vi "DataLog Merge Times.vi"(0 "times to add":dbl[](array[numeric]) format="%<%H:%M:%S%2u\n%Y/%m/%d>T", 7 "times in":dbl[](array[numeric]) format="%<%H:%M:%S%2u\n%Y/%m/%d>T", 11 "error in (no error)":errorcluster) -> (8 "times out":dbl[](array[numeric]) format="%<%H:%M:%S%2u\n%Y/%m/%d>T", 15 "error out":errorcluster)   [LabVIEW 2012]
doc: "Merge times for interpolation. Given two arrays of monotonically increasing times, output an array of times that contains the monotonically increasing union of the input times. When the time arrays contain identical values, the value is copied only once into the output array.\n\nBeware that when either set of times does not increase monotonically, the output times will not either. Though sorting the times is not difficult, this option was rejected to ensure that the algorithm executes in linear time: the arrays might be very large."
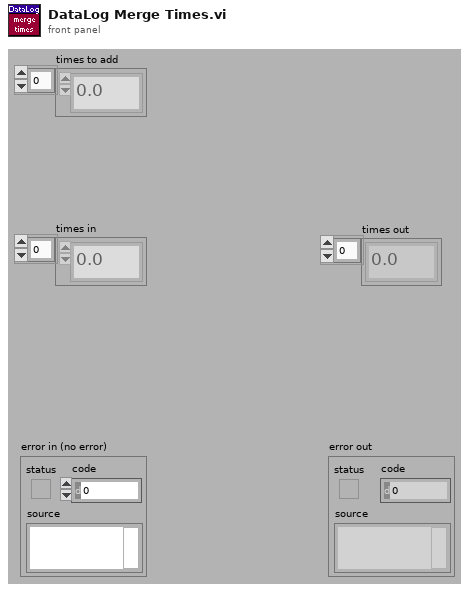
[diagram p1: front panel]
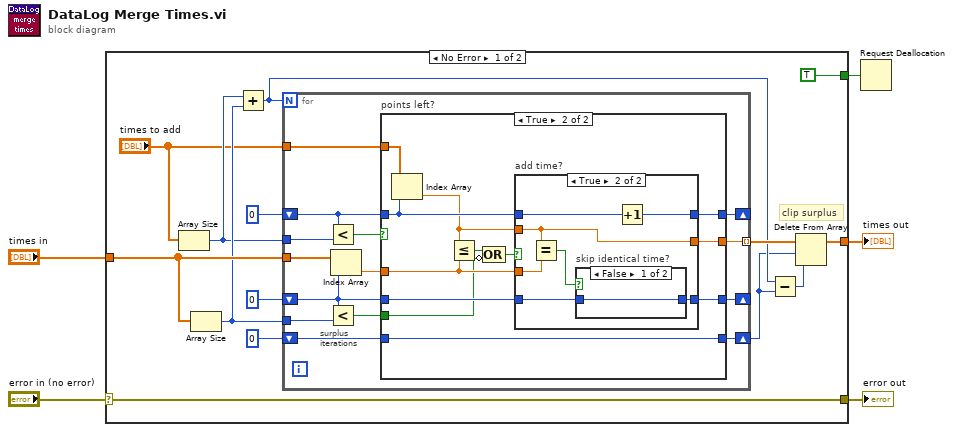
[diagram p0: block diagram]
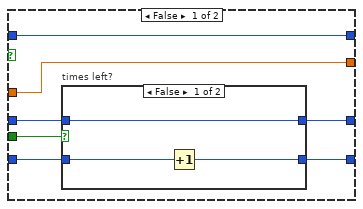
[diagram p2: hidden frame]
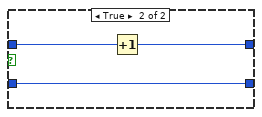
[diagram p3: hidden frame]
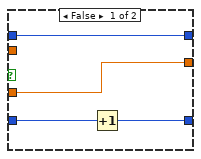
[diagram p4: hidden frame]
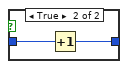
[diagram p5: hidden frame]
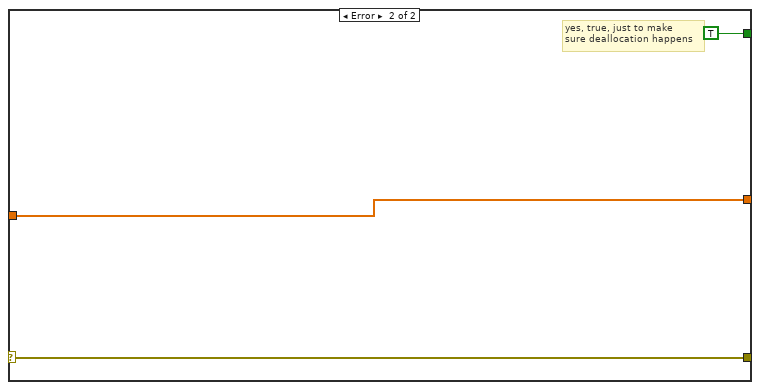
[diagram p6: hidden frame]
diagram:
  n1 = case shown="No Error" "error in (no error)" {
    selector: "error in (no error)" -> [w19 w75]
    tunnel: [w19 w75] -> w4
    tunnel: "times in" -> [w17 w74]
    tunnel: [w16 w74] -> w2
    tunnel: [TRUE ("flag") TRUE ("flag")] -> w1
    frame No Error {
      # "clip surplus"
      n2 = Array Size(array="times to add") -> (size(s)=w7:i32)
      n3 = Array Size(array=w17) -> (size(s)=w8:i32)
      n4 = Add(x=w7, y=w8) -> (x+y=w11:i32)
      n5 = for {
        N: w11 -> [_]
        tunnel: w17 -> [w33]
        tunnel: [w32] -> w15 mode=indexing
        shift-right: [w28] -> _
        shift-left: 0 -> [w25]
        shift-right: [w29] -> _
        shift-left: 0 -> [w21]
        shift-right: [w26] -> w10
        shift-left: 0 -> [w27]
        tunnel: w8 -> [w24]
        tunnel: w7 -> [w22]
        tunnel: "times to add" -> [w30]
        # "surplus\niterations"
        n6 = Less?(x=w21, y=w22) -> (x < y?=w20:bool)
        n7 = Less?(x=w25, y=w24) -> (x < y?=w23:bool)
        n8 = Index Array(array=w33, index=w25) -> (element=w31:dbl)
        n9 = case "points left?" shown="True" w20 {
          tunnel: [w34 w58] -> w32
          tunnel: w31 -> [w34 w57]
          tunnel: w30 -> [_ w52]
          tunnel: w21 -> [w40 w56]
          tunnel: [w40 w55] -> w29
          tunnel: [w37 w54] -> w28
          tunnel: w27 -> [w36 w48]
          tunnel: [w35 w48] -> w26
          tunnel: w25 -> [w38 w53]
          tunnel: w23 -> [w39 w50]
          frame False {
            n10 = case "times left?" shown="False" w39 {
              tunnel: w38 -> [w41 w46]
              tunnel: [w41 w45] -> w37
              tunnel: w36 -> [w43 w44]
              tunnel: [w42 w44] -> w35
              frame False {
                n11 = Increment(x=w43) -> (x+1=w42:i32)
              }
              frame True {
                n12 = Increment(x=w46) -> (x+1=w45:i32)
              }
            }
          }
          frame True {
            n13 = Index Array(array=w52, index=w56) -> (element=w47:dbl)
            n14 = Less Or Equal?(x=w47, y=w57) -> (x <= y?=w51:bool)
            n15 = Compound Arithmetic op=OR(w51, invert w50) -> (w49:bool)
            n16 = case "add time?" shown="True" w49 {
              tunnel: [w62 w68] -> w58
              tunnel: w57 -> [w62 w69]
              tunnel: w47 -> [_ w68]
              tunnel: [w61 w66] -> w55
              tunnel: w56 -> [w61 w67]
              tunnel: w53 -> [w60 w64]
              tunnel: [w59 w63] -> w54
              frame False {
                n17 = Increment(x=w60) -> (x+1=w59:i32)
              }
              frame True {
                n18 = Equal?(x=w68, y=w69) -> (x = y?=w65:bool)
                n19 = case "skip identical time?" shown="False" w65 {
                  tunnel: w64 -> [w70 w72]
                  tunnel: [w70 w71] -> w63
                  frame False {
                  }
                  frame True {
                    n20 = Increment(x=w72) -> (x+1=w71:i32)
                  }
                }
                n21 = Increment(x=w67) -> (x+1=w66:i32)
              }
            }
          }
        }
      }
      n22 = Subtract(x=w11, y=w10) -> (x-y=w9:i32)
      n23 = Delete From Array(array=w15, length=w10, index=w9) -> (array with subset deleted=w16:dbl[])  [unwired: 1 out]
    }
    frame Error {
      # "yes, true, just to make\nsure deallocation happens"
    }
  }
  "times out" <- w2
  "error out" <- w4
  n24 = Request Deallocation(w1) -> ()
